vi "sensor2numeric.vi"(0 "Sensor4(MSB)":bool, 2 "Sensor3":bool, 4 "Sensor2":bool, 9 "Sensor1":bool, 13 "Sensor0(LSB)":bool) -> (14 "Numeric":dbl)   [LabVIEW 2011]
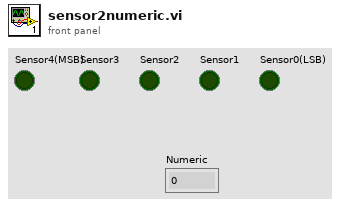
[diagram p1: front panel]
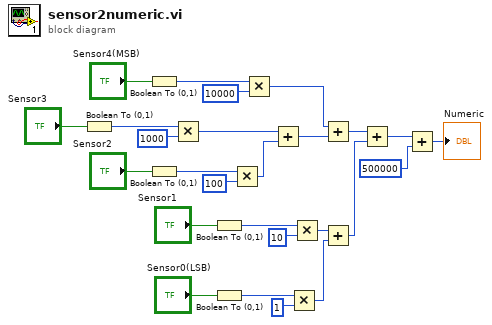
[diagram p0: block diagram]
diagram:
  n1 = Boolean To (0,1)(Boolean="Sensor3") -> (0, 1=w11:i16)
  n2 = Boolean To (0,1)(Boolean="Sensor4(MSB)") -> (0, 1=w10:i16)
  n3 = Boolean To (0,1)(Boolean="Sensor2") -> (0, 1=w6:i16)
  n4 = Multiply(x=w11, y=1000) -> (x*y=w23:i32)
  n5 = Boolean To (0,1)(Boolean="Sensor1") -> (0, 1=w4:i16)
  n6 = Boolean To (0,1)(Boolean="Sensor0(LSB)") -> (0, 1=w12:i16)
  n7 = Multiply(x=w6, y=100) -> (x*y=w24:i32)
  n8 = Multiply(x=w10, y=10000) -> (x*y=w22:i32)
  n9 = Add(x=w23, y=w24) -> (x+y=w21:i32)
  n10 = Multiply(x=w12, y=1) -> (x*y=w26:i32)
  n11 = Multiply(x=w4, y=10) -> (x*y=w25:i32)
  n12 = Add(x=w22, y=w21) -> (x+y=w20:i32)
  n13 = Add(x=w25, y=w26) -> (x+y=w19:i32)
  n14 = Add(x=w20, y=w19) -> (x+y=w3:i32)
  n15 = Add(x=w3, y=500000) -> (x+y=→"Numeric":i32)
